vi "Launcher.vi"() -> ()   [LabVIEW 2024]
uses:
  <vilib>/Utility/miscctls.llb/LVRectTypeDef.ctl
  CarFactory/CarFactory.lvclass
  ICarProduct/ICarProduct.lvclass
panel:
  in  "Close Button":bool
  out "CarType":string
  in  "Car Types":string(combo)
  in  "Create Car":bool
  out "Car Picture":picture
  # "Car Type"
  # "Car Type"
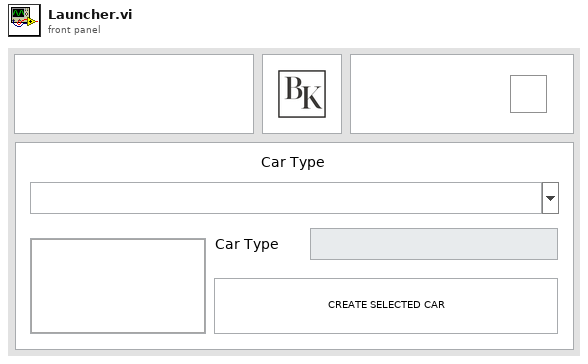
[diagram p1: front panel]
types:
  T1 = typedef "LVRectTypeDef.ctl" = cluster{"Left":i16, "Top":i16, "Right":i16, "Bottom":i16}
  T2 = typedef "imagedata.ctl" = cluster{"image type":i32, "image depth":i32, "image":u8[], "mask":u8[], "colors":u32[], "Rectangle":cluster{"left":i16, "top":i16, "right":i16, "bottom":i16}}
  T3 = typedef "LVBoundsTypeDef.ctl" = cluster{"Width":u32, "Height":u32}
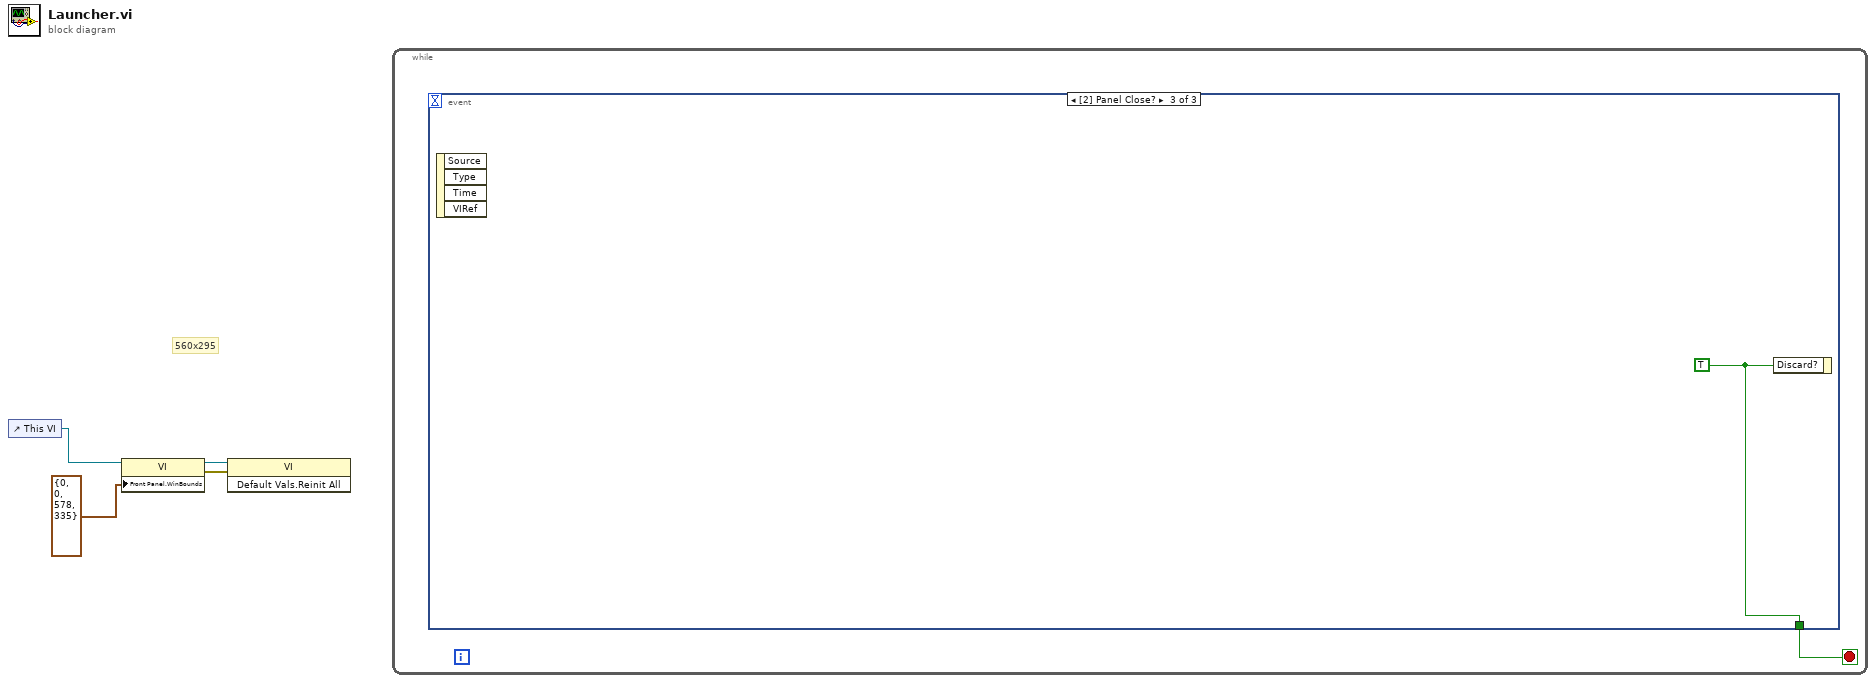
[diagram p0: block diagram]
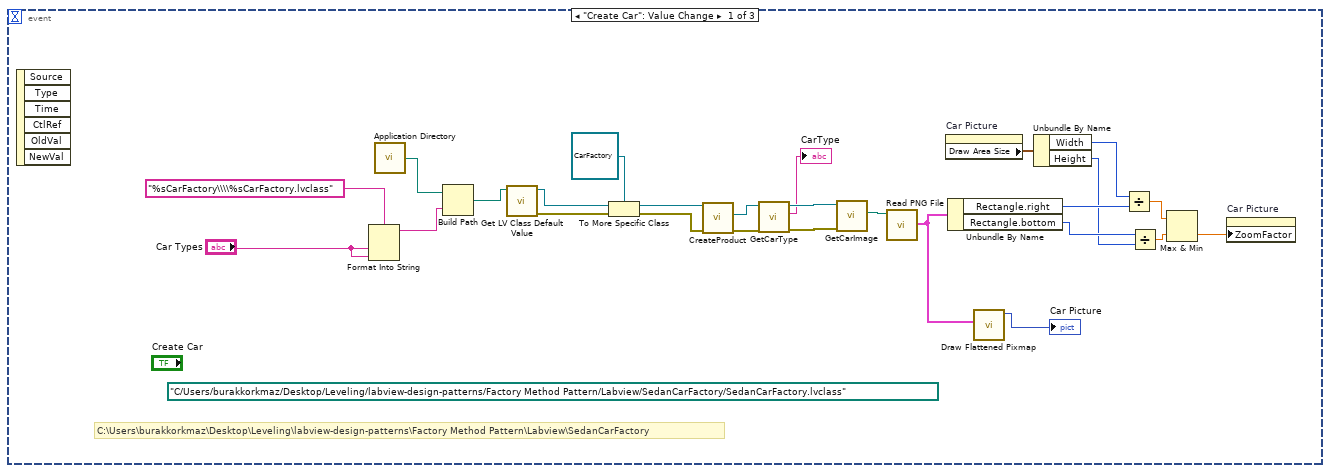
[diagram p2: hidden frame]
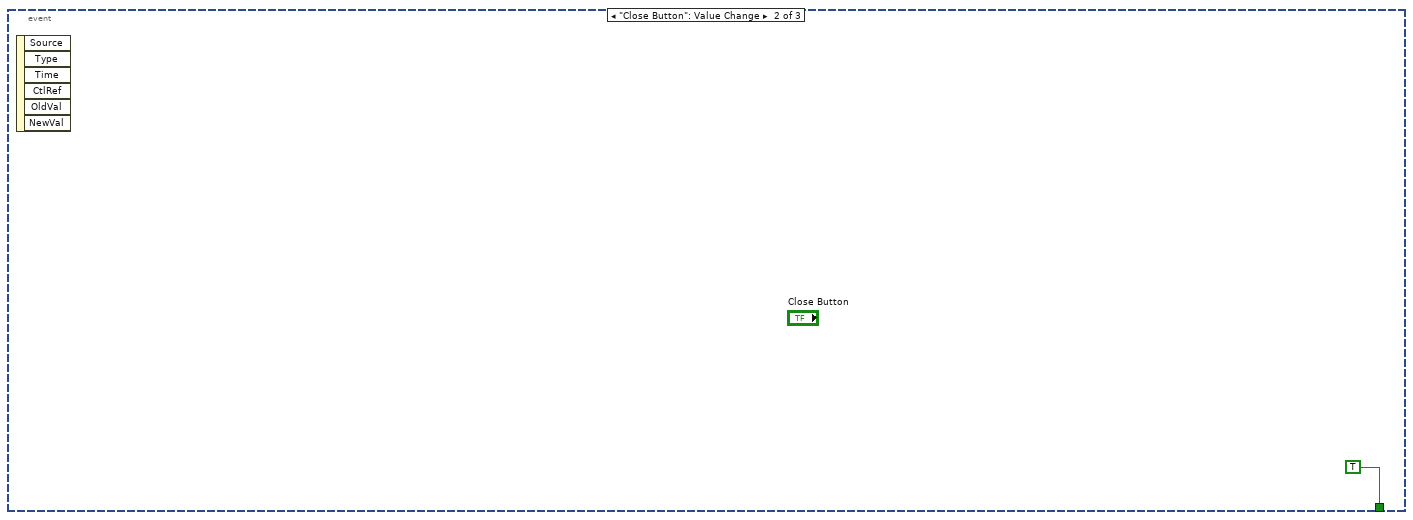
[diagram p3: hidden frame]
diagram:
  # "560x295"
  n1 = control-ref of="This VI"() -> (w4:refnum<vi>)
  n2 = property class="VI"(reference=w4, "Front Panel.WinBounds"=T1 {"Left"=0, "Top"=0, "Right"=578, "Bottom"=335} ("Front Panel Window:Window Bounds")) -> (reference out=w2:refnum<vi>, error out=w1:errorcluster)  [unwired: 1 in]
  n3 = invoke class="VI" method="Default Vals.Reinit All"(reference=w2, error in=w1) -> ()  [unwired: 1 in, 3 out]
  n4 = while {
    stop <- w5 stop-if-true
    n5 = event shown="[2] Panel Close?" {
      selector: _ -> [_ _ _]
      dyn-events: _ -> [_ _ _]
      timeout: _ -> [_ _ _]
      tunnel: [_ TRUE w33] -> w5
      event "Create Car": Value Change {
        (unwired) path "C:/Users/burakkorkmaz/Desktop/Leveling/labview-design-patterns/Factory Method Pattern/Labview/SedanCarFactory/SedanCarFactory.lvclass"
        # "C:\\Users\\burakkorkmaz\\Desktop\\Leveling\\labview-design-patterns\\Factory Method Pattern\\Labview\\SedanCarFactory"
        n6 = event-data() -> ()  [unwired: 1 in, 6 out]
        n7 = Format Into String(format string="%sCarFactory\\\\%sCarFactory.lvclass", "Car Types", "Car Types") -> (resulting string=w9:string)  [unwired: 2 in, 1 out]
        n8 = call <vilib>:"Application Directory.vi"() -> ("Application Directory"=w31:path)
        n9 = Build Path(base path=w31, name or relative path=w9) -> (appended path=w8:path)
        n10 = call <vilib>:"Get LV Class Default Value.vi"("class path"=w8) -> ("error out"=w29:errorcluster, "object"=w30:refnum<class>)  [unwired: 9 in]
        n11 = To More Specific Class(target class=refnum<class "CarFactory.lvclass"> refnum ("CarFactory"), reference=w30, error in=w29) -> (specific class reference=w25:refnum<class "CarFactory.lvclass">, error out=w26:errorcluster)
        n12 = call-dynamic "CreateProduct.vi"("Error In"=w26, "reference in"=w25) -> ("Error Out"=w27:errorcluster, "ICarProduct"=w28:refnum<class "ICarProduct.lvclass">)  [unwired: 7 in, 1 out]
        n13 = call-dynamic "GetCarType.vi"("Error In"=w27, "object in"=w28) -> ("Error Out"=w23:errorcluster, "Car Type"=→"CarType":string, "object out"=w22:refnum<class "ICarProduct.lvclass">)  [unwired: 7 in]
        n14 = call-dynamic "GetCarImage.vi"("Error In"=w23, "object in"=w22) -> ("Image Path"=w20:path)  [unwired: 7 in, 2 out]
        n15 = call <vilib>:"Read PNG File.vi"("path to PNG file"=w20) -> ("image data"=w13:T2)  [unwired: 8 in, 2 out]
        n16 = property on="Car Picture" class="Pict"() -> ("Draw Area Size"=w19:T3)  [unwired: 2 in, 2 out]
        n17 = Unbundle By Name(w13) -> ("Rectangle.right"=w18:i16, "Rectangle.bottom"=w17:i16)
        n18 = call <vilib>:"Draw Flattened Pixmap.vi"("image data"=w13) -> ("new picture"=→"Car Picture":picture)  [unwired: 8 in]
        n19 = Unbundle By Name(w19) -> ("Width"=w7:u32, "Height"=w6:u32)
        n20 = Divide(x=w7, y=w18) -> (x/y=w15:dbl)
        n21 = Divide(x=w17, y=w6) -> (x/y=w16:dbl)
        n22 = Max & Min(x=w15, y=w16) -> (min(x,y)=w14:dbl)  [unwired: 1 out]
        n23 = property on="Car Picture" class="Pict"("ZoomFactor"=w14) -> ()  [unwired: 2 in, 2 out]
      }
      event "Close Button": Value Change {
        n24 = event-data() -> ()  [unwired: 1 in, 6 out]
      }
      event Panel Close? {
        w33 = TRUE ("Discard?")
        n25 = event-data() -> ()  [unwired: 1 in, 4 out]
        n26 = event-data("Discard?"=w33) -> ()  [unwired: 1 in, 1 out]
      }
    }
  }
